vi "get_LM_IDs_by_name.vi"(8 "error in (no error)":errorcluster caption="错误输入（无错误）", 10 "name":string, 11 "MotorSystem 输入":refnum<class "MotorSystem.lvclass">) -> (0 "error out":errorcluster caption="错误输出", 2 "簇":cluster{"LM ID -":T1, "LM ID +":T1}={"LM ID -"=1, "LM ID +"=1} {"LM ID +" items=["none", "S1", "S2", "S3"]; "LM ID -" items=["none", "S1", "S2", "S3"]}, 3 "MotorSystem 输出":refnum<class "MotorSystem.lvclass">)   [LabVIEW 2016, in "MotionControl.lvlib" / "MotorSystem.lvclass"]
uses:
  <userlib>/MotionControl/MotorSystem/MotorSystem.lvclass
  <userlib>/MotionControl/LimitSwitch/LM_ID.ctl
  <userlib>/MotionControl/MotorSystem/MotorSystem.lvclass/MotorSystem.ctl
  <userlib>/MotionControl/OneMotion/OneMotion.lvclass/OneMotion.ctl
  <userlib>/MotionControl/LimitSwitch/LimitSwitch.lvclass/LimitSwitch.ctl
  <userlib>/MotionControl/OneMotion/OneMotion.lvclass
  <userlib>/MotionControl/LimitSwitch/LimitSwitch.lvclass
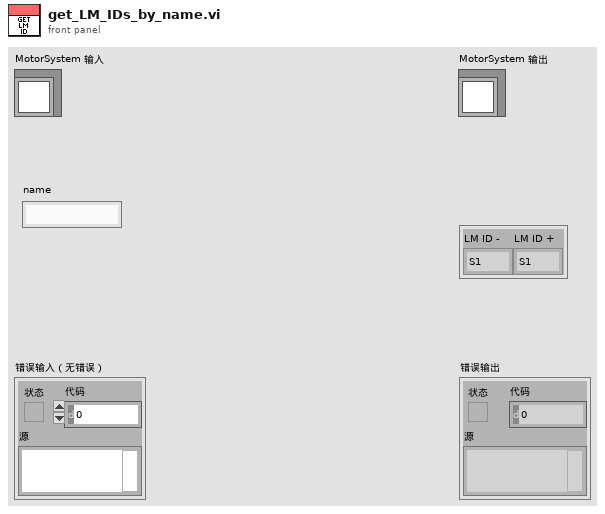
[diagram p1: front panel]
types:
  T1 = typedef "MotionControl.lvlib/LimitSwitch.lvclass/LM_ID.ctl" = i32
  T2 = typedef "MotionControl.lvlib/MotorSystem.lvclass/MotionCluster.ctl" = cluster{"OneMotion.lvclass":refnum<class "OneMotion.lvclass">, "connected?":bool, "default enabled?":bool, "enabled?":bool}
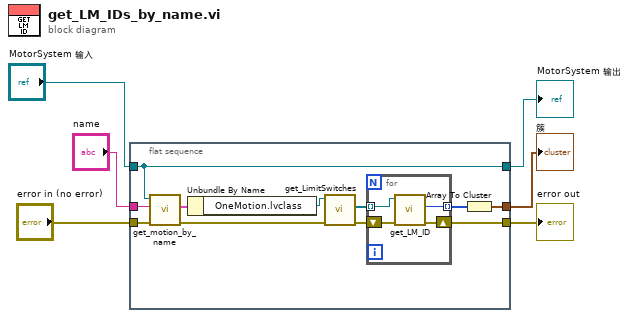
[diagram p0: block diagram]
diagram:
  n1 = flat-sequence {
    tunnel: [w9] -> w6
    tunnel: [w17] -> w4
    tunnel: "MotorSystem 输入" -> [w17]
    tunnel: "error in (no error)" -> [w15]
    tunnel: [w7] -> w1
    tunnel: "name" -> [w16]
    frame #0 {
      n2 = call <userlib>:"get_motion_by_name.vi"("error in (no error)"=w15, "name"=w16, "MotorSystem in"=w17) -> ("error out"=w14:errorcluster, "motion cluster"=w11:T2)  [unwired: 6 in, 1 out]
      n3 = Unbundle By Name(w11) -> ("OneMotion.lvclass"=w13:refnum<class "OneMotion.lvclass">)
      n4 = call <userlib>:"get_LimitSwitches.vi"("error in (no error)"=w14, "OneMotion输入"=w13) -> ("error out"=w12:errorcluster, "LimitSwitches"=w10:refnum<class "LimitSwitch.lvclass">[])  [unwired: 7 in, 1 out]
      n5 = for {
        tunnel: [w21] -> w8 mode=indexing
        shift-right: [w19] -> w9
        shift-left: w12 -> [w20]
        tunnel: w10 -> [w18] mode=indexing
        n6 = call <userlib>:"get_LM_ID.vi"("error in (no error)"=w20, "LimitSwitch输入"=w18) -> ("error out"=w19:errorcluster, "LM ID"=w21:T1)  [unwired: 7 in, 1 out]
      }
      n7 = Array To Cluster(array=w8) -> (cluster=w7:cluster{"[0]":T1, "[1]":T1})
    }
  }
  "error out" <- w6
  "MotorSystem 输出" <- w4
  "簇" <- w1
